vi "Reorder Array Increasing.vi"(9 "Make decremental?":bool, 10 "X row":i32, 11 "Array":dbl[][](array[numeric])) -> (3 "Output array":dbl[][](array[numeric]))   [LabVIEW 2024]
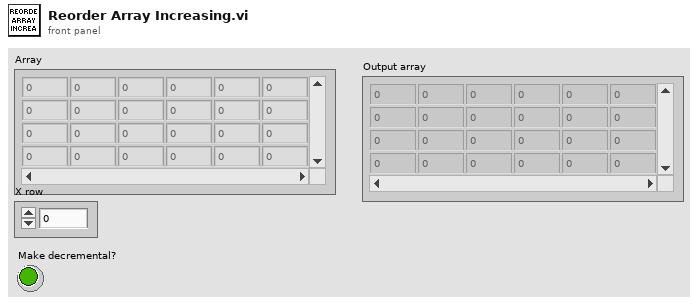
[diagram p1: front panel]
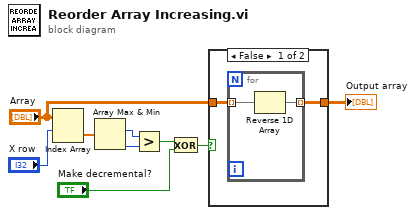
[diagram p0: block diagram]
diagram:
  n1 = Index Array(array="Array", index (row)="X row") -> (element=w3:dbl[])  [unwired: 1 in]
  n2 = Array Max & Min(array=w3) -> (max index (indices)=w8:i32, min index (indices)=w7:i32)  [unwired: 2 out]
  n3 = Greater?(x=w8, y=w7) -> (0:w6:bool)
  n4 = Exclusive Or(1:"Make decremental?", 2:w6) -> (0:w4:bool)
  n5 = case shown="False" w4 {
    tunnel: "Array" -> [w11 w14]
    tunnel: [w10 w14] -> w1
    frame False {
      n6 = for {
        tunnel: w11 -> [w13] mode=indexing
        tunnel: [w12] -> w10 mode=indexing
        n7 = Reverse 1D Array(array=w13) -> (reversed array=w12:dbl[])
      }
    }
    frame True {
    }
  }
  "Output array" <- w1
